vi "剖面运行流程.vi"() -> ()   [LabVIEW 2016, in "main.lvlib"]
uses:
  main.lvlib
  DAM395CF/DAM395CF.lvlib
  elevator/elevator.lvlib
  EXO2/EXO2.lvlib
  bbe/bbe.lvlib
  <vilib>/ptbypt/NI_PtbyPt.lvlib
panel:
  out "监测开始时间":timestamp
  out "编码器校准开始时间":timestamp
  out "仪器启动时间":timestamp
  out "通电时间":timestamp
  in  "bbe data":T1[](array[typedef])
  in  "EXO2 data":T2[](array[typedef])
  out "监测数据表":string[][](array[string])
  out "最深位置":dbl
  out "通知":bool
  out "Next State":string
  out "剖面路径":dbl[](array[numeric])
  out "湖面水深":dbl format="%#_6f m"
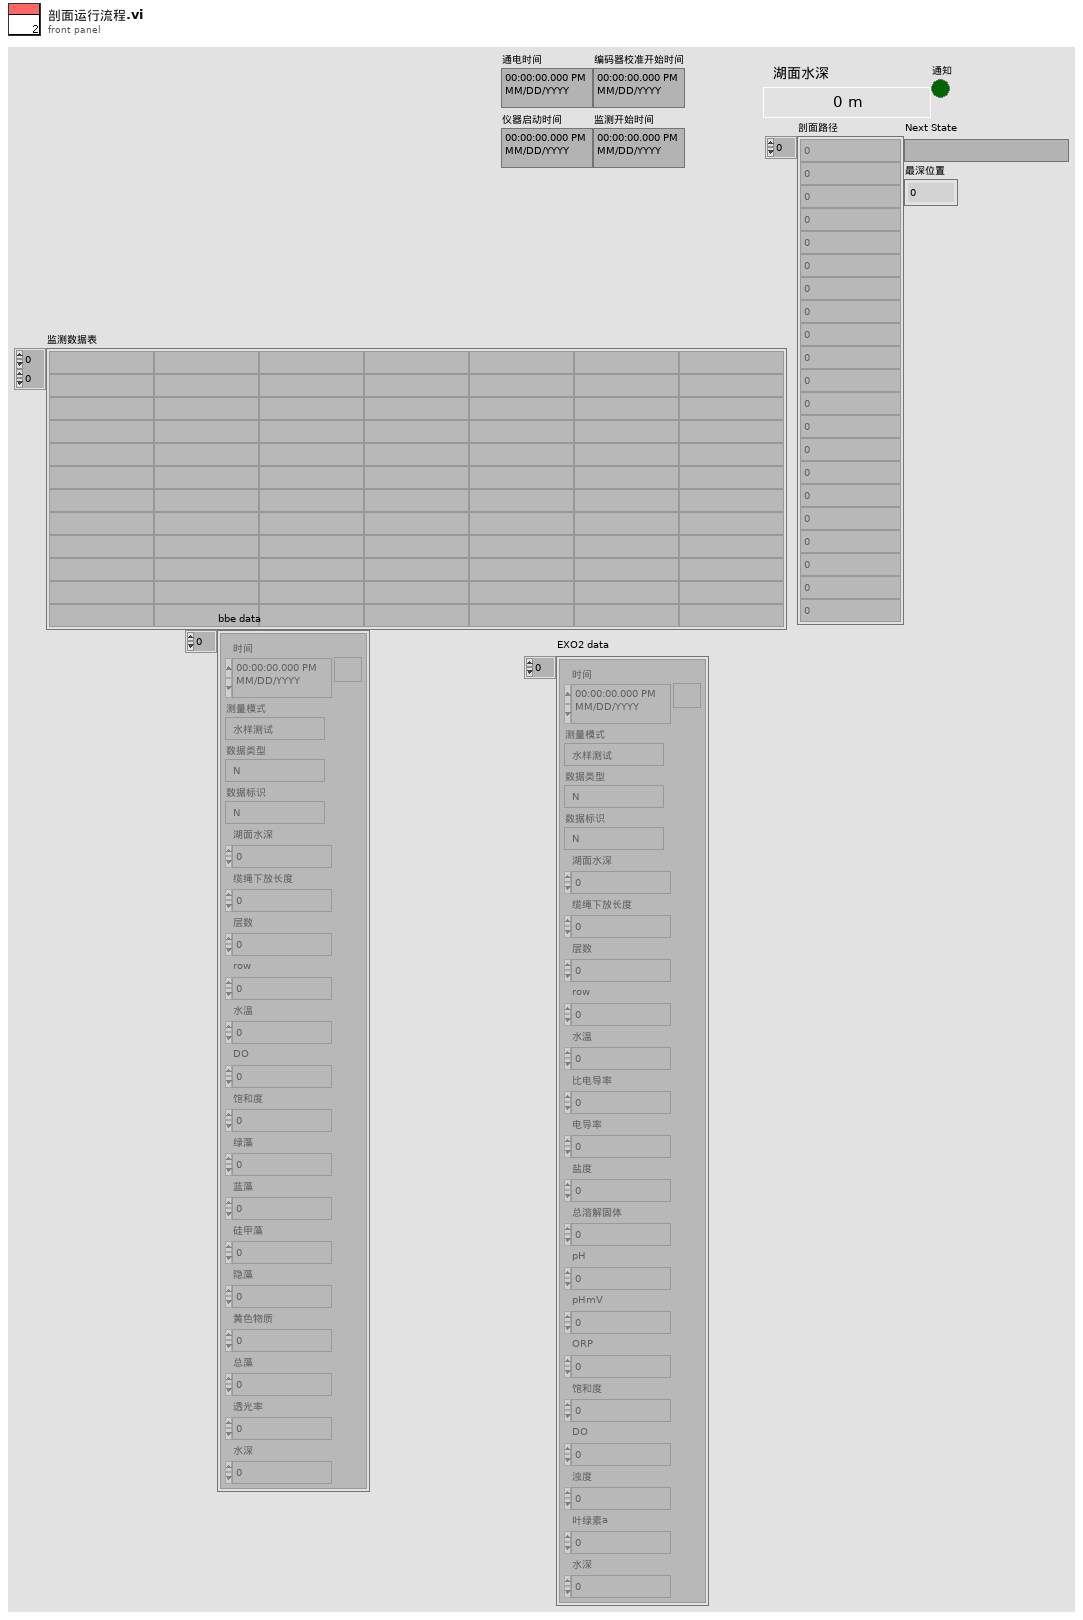
[diagram p1: front panel]
types:
  T1 = typedef "剖面数据_bbe_NAQDO.ctl" = cluster{"时间":timestamp, "测量模式":string, "数据类型":string, "数据标识":string, "湖面水深":sgl, "缆绳下放长度":sgl, "层数":u16, "row":u16, "水温":sgl, "DO":sgl, "饱和度":sgl, "绿藻":sgl, "蓝藻":sgl, "硅甲藻":sgl, "隐藻":sgl, "黄色物质":sgl, "总藻":sgl, "透光率":sgl, "水深":sgl}
  T2 = typedef "剖面数据_EXO2.ctl" = cluster{"时间":timestamp, "测量模式":string, "数据类型":string, "数据标识":string, "湖面水深":sgl, "缆绳下放长度":sgl, "层数":u16, "row":u16, "水温":sgl, "比电导率":sgl, "电导率":sgl, "盐度":sgl, "总溶解固体":sgl, "pH":sgl, "pHmV":sgl, "ORP":sgl, "饱和度":sgl, "DO":sgl, "浊度":sgl, "叶绿素a":sgl, "水深":sgl}
  T3 = enum16{"open", "poll", "close", "run", "stop", "shutdown"}
  T4 = typedef "操作日志字段定义.ctl" = cluster{"时间":timestamp, "参数":string, "日志信息":string, "流程参数":string}
  T5 = cluster{"Time":timestamp, "Temp":dbl, "SpCond":dbl, "Cond":dbl, "Sal":dbl, "TDS":dbl, "pH":dbl, "pH mV":dbl, "orp":dbl, "ODO %":dbl, "ODO mg/L":dbl, "Turb":dbl, "Chl":dbl, "Depth":dbl}
  T6 = cluster{"时间":timestamp, "Temp [℃]":dbl, "Green Algae [μg/L]":dbl, "Bluegreen [μg/L]":dbl, "Diatoms [μg/L]":dbl, "Cryptophyta [μg/L]":dbl, "Yellow substances [r.u.]":dbl, "Total Conc [μg/L]":dbl, "Transmission [%]":dbl, "Depth [m]":dbl}
  T7 = cluster{"水温":sgl, "比电导率":sgl, "电导率":sgl, "盐度":sgl, "总溶解固体":sgl, "pH":sgl, "pHmV":sgl, "ORP":sgl, "饱和度":sgl, "DO":sgl, "浊度":sgl, "叶绿素a":sgl, "水深":sgl}
  T8 = cluster{"水温":sgl, "DO":sgl, "饱和度":sgl, "绿藻":sgl, "蓝藻":sgl, "硅甲藻":sgl, "隐藻":sgl, "黄色物质":sgl, "总藻":sgl, "透光率":sgl, "水深":sgl}
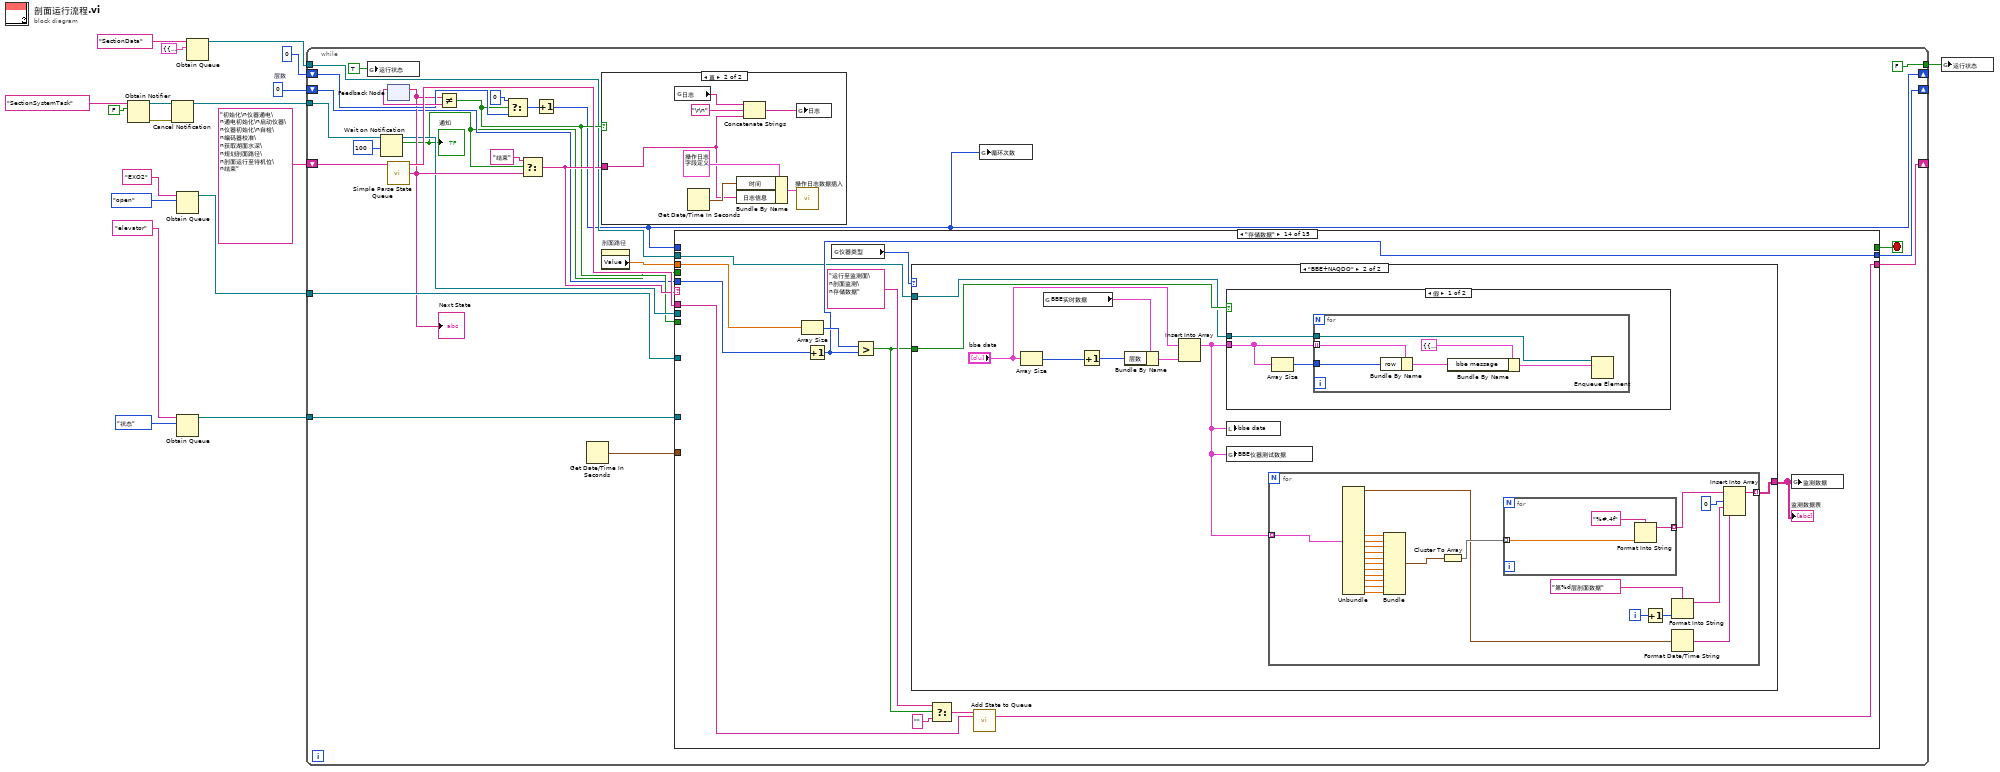
[diagram p0: block diagram]
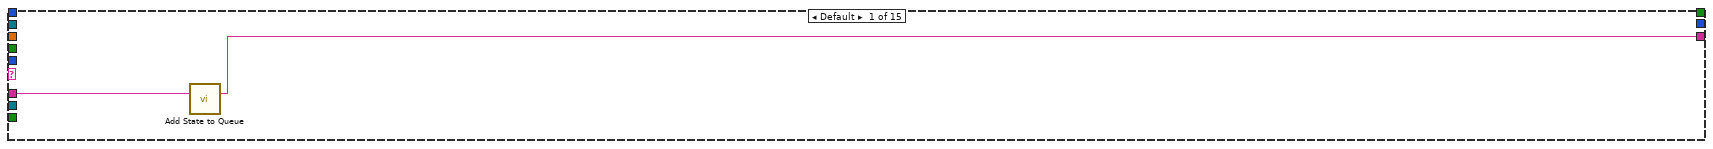
[diagram p3: hidden frame]
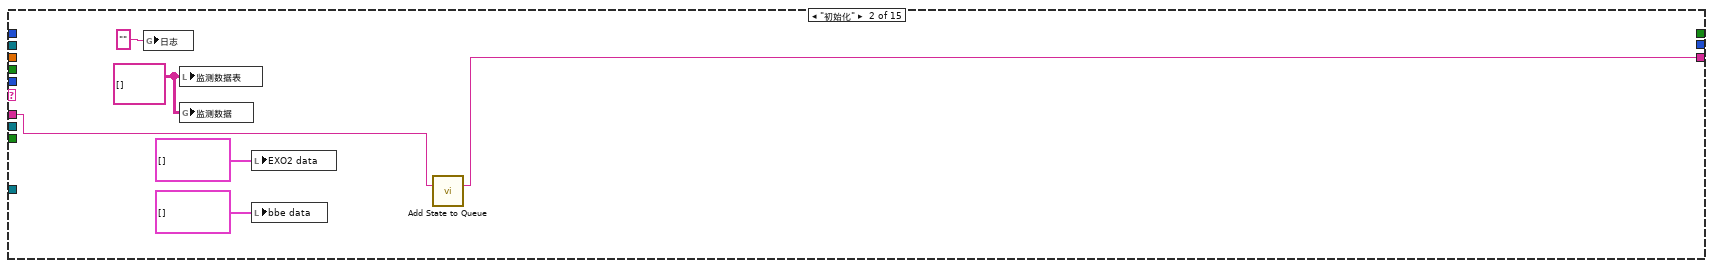
[diagram p4: hidden frame]
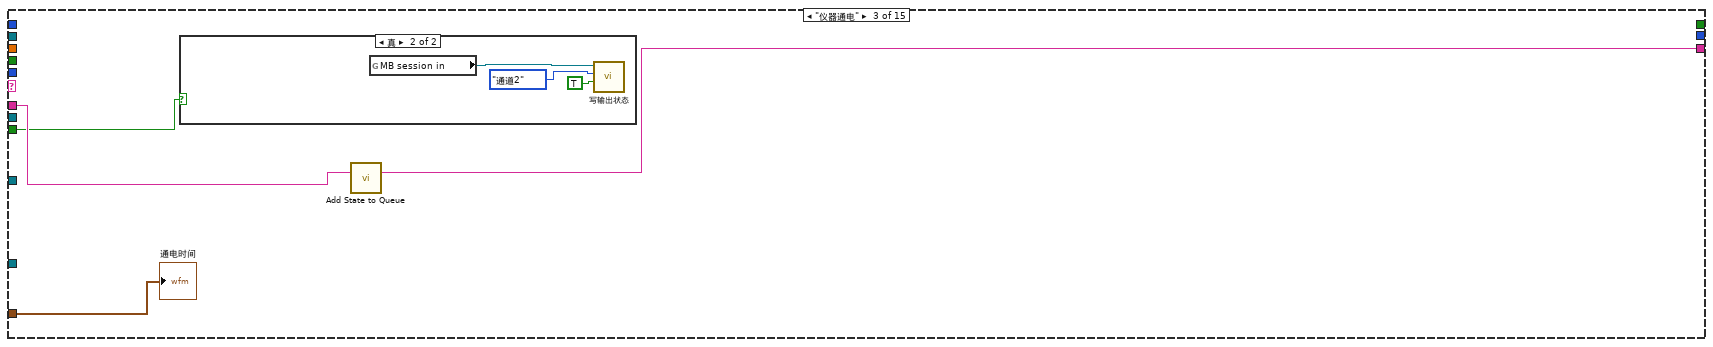
[diagram p5: hidden frame]
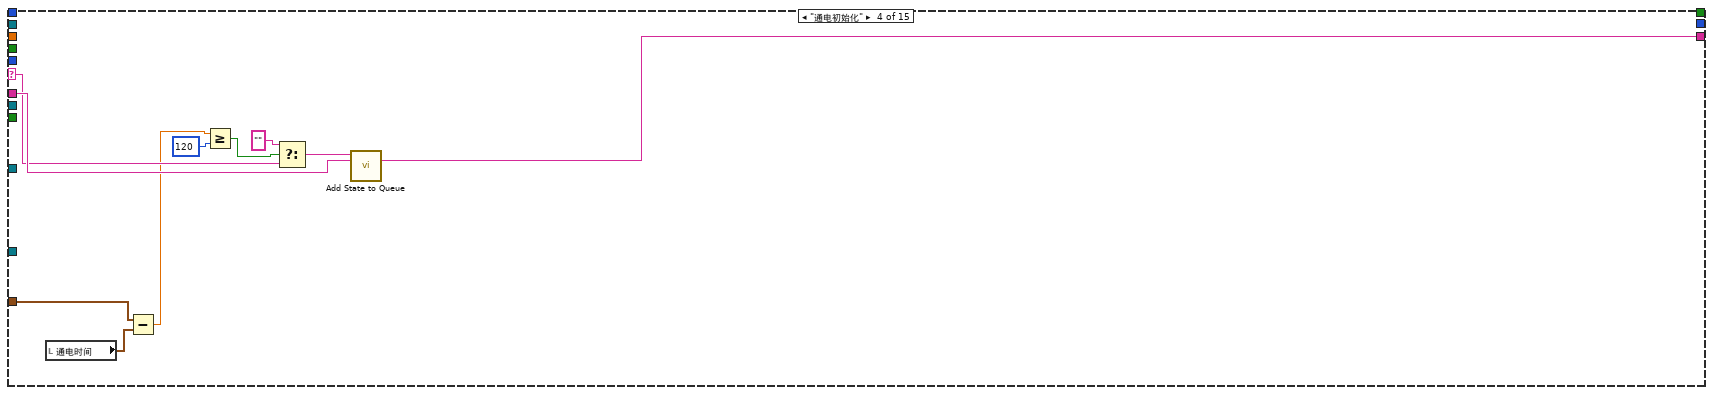
[diagram p7: hidden frame]
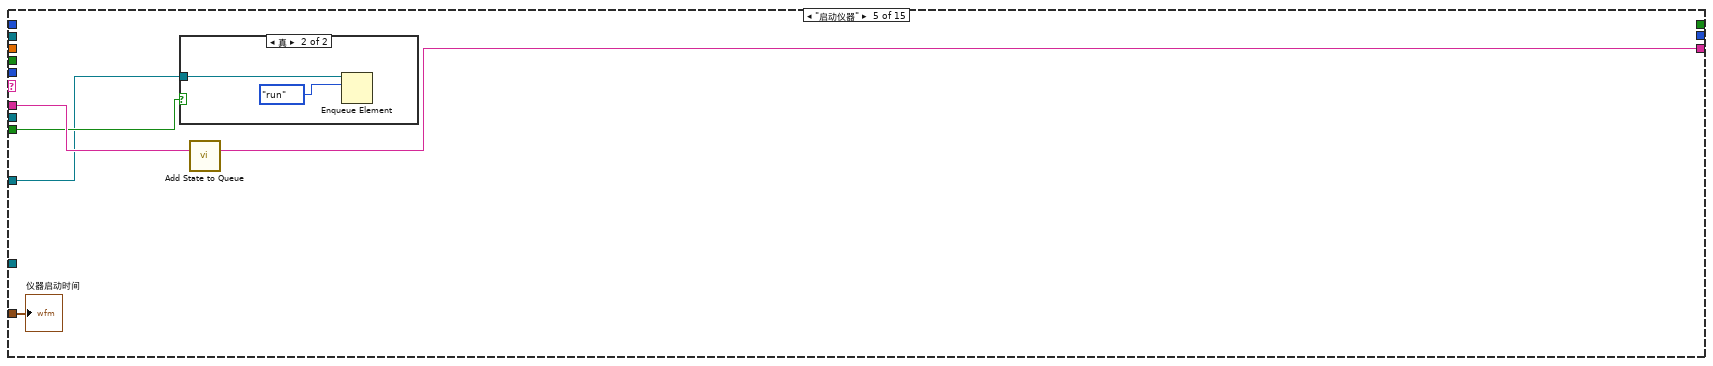
[diagram p8: hidden frame]
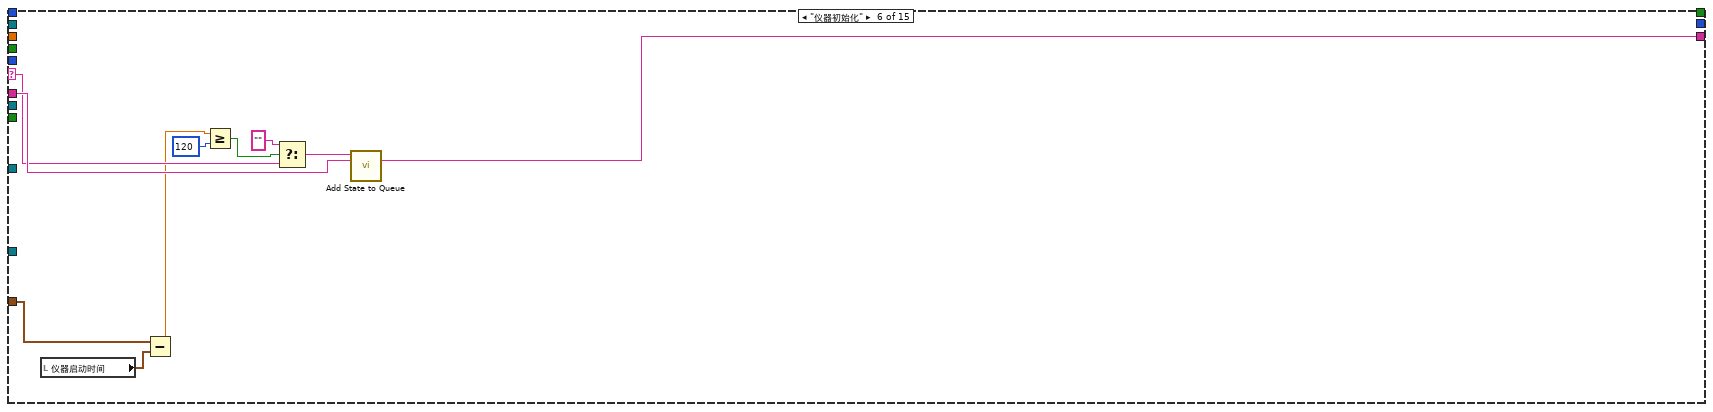
[diagram p10: hidden frame]
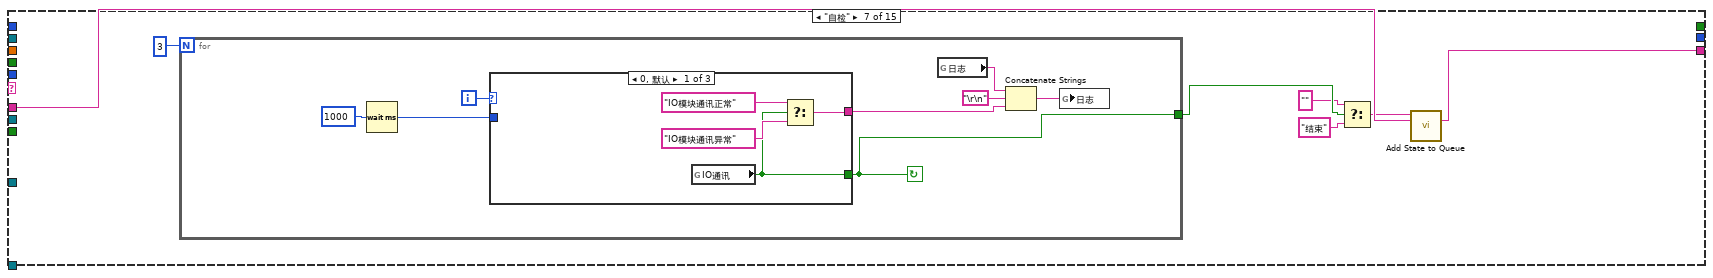
[diagram p11: hidden frame]
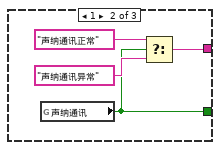
[diagram p12: hidden frame]
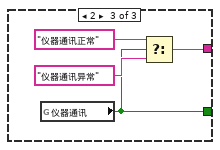
[diagram p13: hidden frame]
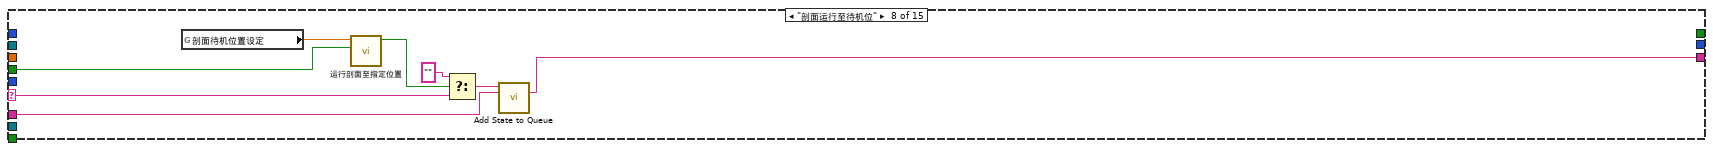
[diagram p14: hidden frame]
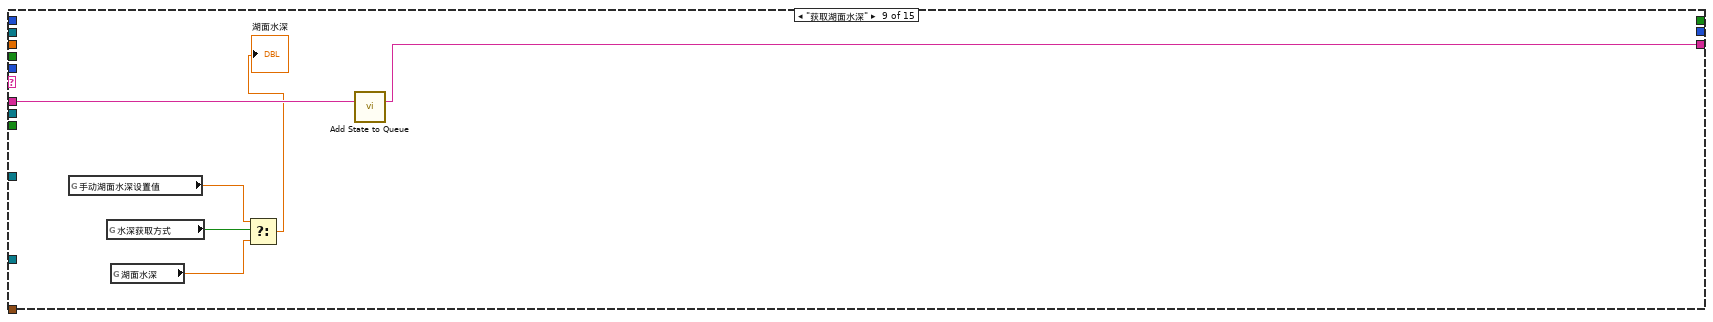
[diagram p15: hidden frame]
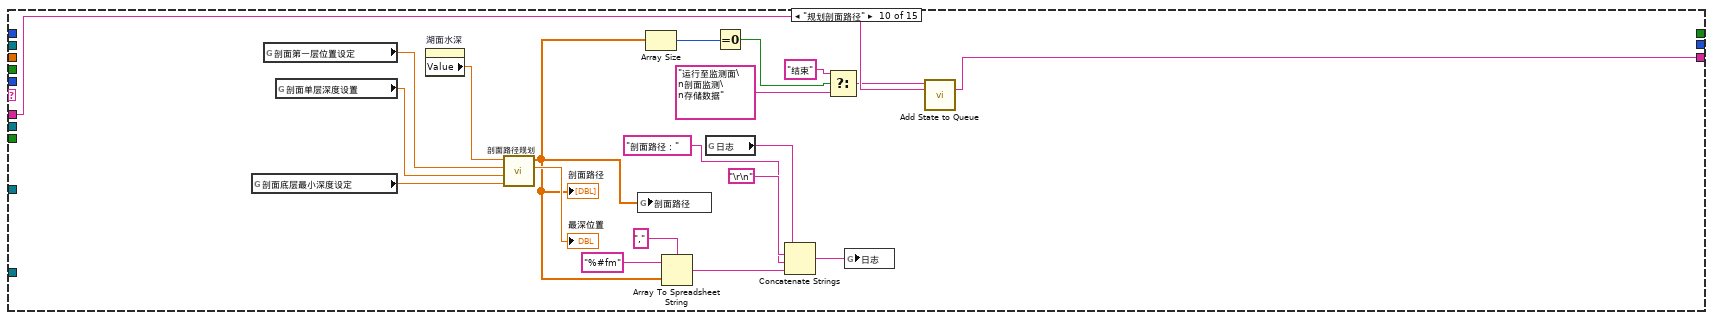
[diagram p16: hidden frame]
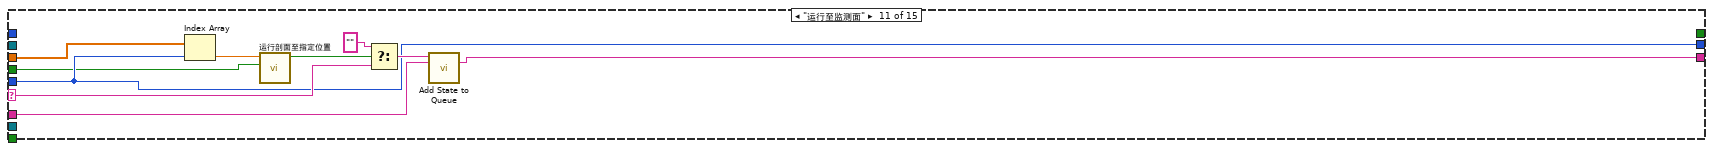
[diagram p17: hidden frame]
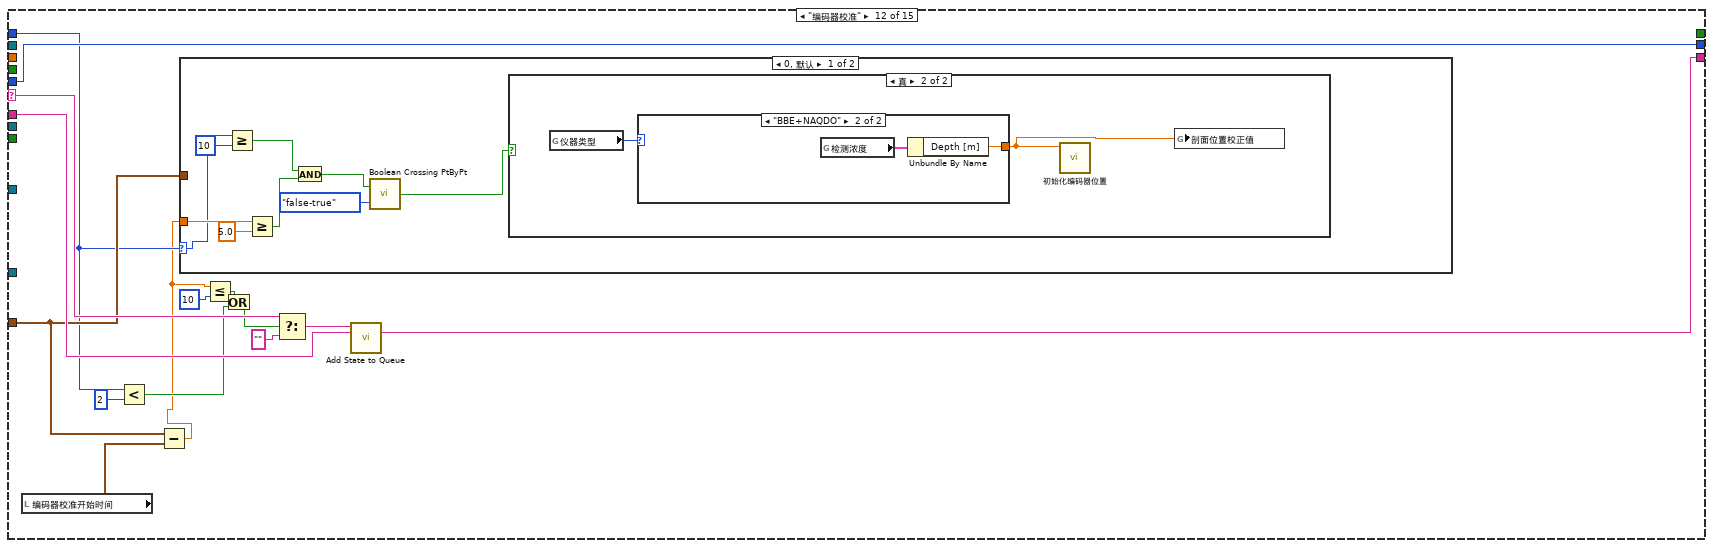
[diagram p18: hidden frame]
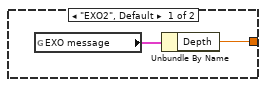
[diagram p20: hidden frame]
diagram:
  w5 = 0  # 层数
  n1 = Obtain Notifier(name (unnamed)="SectionSystemTask" ("名称（未命名）"), notification data type=FALSE) -> (notifier out=w7:refnum<notifier>, error out=w8:errorcluster)  [unwired: 2 in, 1 out]
  n2 = Cancel Notification(0:w7, 3:w8) -> (8:w6:refnum<notifier>)  [unwired: 2 out]
  n3 = Obtain Queue(name (unnamed)="EXO2" ("名称（未命名）"), element data type=T3."open" ("枚举")) -> (queue out=w12:refnum<queue>)  [unwired: 3 in, 2 out]
  n4 = Obtain Queue(name (unnamed)="elevator" ("名称（未命名）"), element data type=enum16{"状态", "上升", "下降", "停止"}."状态" ("枚举")) -> (queue out=w11:refnum<queue>)  [unwired: 3 in, 2 out]
  n5 = Obtain Queue(name (unnamed)="SectionData" ("名称（未命名）"), element data type=cluster{"EXO2 message":T2, "bbe message":T1} {"EXO2 message"={"时间"=timestamp(0 s since 1904-01-01), "测量模式"="水样测试", "数据类型"="N", "数据标识"="N", "湖面水深"=0.0, "缆绳下放长度"=0.0, "层数"=0, "row"=0, "水温"=0.0, "比电导率"=0.0, "电导率"=0.0, "盐度"=0.0, "总溶解固体"=0.0, "pH"=0.0, "pHmV"=0.0, "ORP"=0.0, "饱和度"=0.0, "DO"=0.0, "浊度"=0.0, "叶绿素a"=0.0, "水深"=0.0}, "bbe message"={"时间"=timestamp(0 s since 1904-01-01), "测量模式"="水样测试", "数据类型"="N", "数据标识"="N", "湖面水深"=0.0, "缆绳下放长度"=0.0, "层数"=0, "row"=0, "水温"=0.0, "DO"=0.0, "饱和度"=0.0, "绿藻"=0.0, "蓝藻"=0.0, "硅甲藻"=0.0, "隐藻"=0.0, "黄色物质"=0.0, "总藻"=0.0, "透光率"=0.0, "水深"=0.0}} ("簇")) -> (queue out=w2:refnum<queue>)  [unwired: 3 in, 2 out]
  n6 = while {
    shift-right: [w43] -> _
    shift-left: "初始化\n仪器通电\n通电初始化\n启动仪器\n仪器初始化\n自检\n编码器校准\n获取湖面水深\n规划剖面路径\n剖面运行至待机位\n结束" -> [w44]
    shift-right: [w20] -> _
    shift-left: 0 -> [w39]
    tunnel: w12 -> [w36]
    tunnel: w11 -> [w35]
    tunnel: w6 -> [w34]
    shift-right: [w26] -> _
    shift-left: w5 -> [w27]
    tunnel: [FALSE ("运行状态")] -> w4
    tunnel: w2 -> [w21]
    stop <- w42 stop-if-true
    n7 = global write "全局非断电保持变量.vi" "运行状态"(TRUE ("运行状态")) -> ()
    n8 = Wait on Notification(notifier=w34, timeout in ms (-1)=100 ("超时毫秒(-1)")) -> (notifier out=w30:refnum<notifier>, notification=w22:bool)  [unwired: 2 in, 2 out]
    "通知" <- w22
    n9 = feedback #1() -> (w40:string)  [unwired: 1 in]
    n10 = call "Simple Parse State Queue.vi"("State Queue"=w44) -> ("Remain States"=w41:string, "Next State"=w32:string)  [unwired: 13 in]
    "Next State" <- w32
    n11 = feedback-in #1(w32) -> ()
    n12 = Not Equal?(x=w32, y=w40) -> (x != y?=w28:bool)
    n13 = Select(t=0, s=w28, f=w39) -> (s? t:f=w38:i32)
    n14 = Select(t="结束", s=w22, f=w32) -> (s? t:f=w29:string)
    n15 = Increment(x=w38) -> (x+1=w20:i32)
    n16 = Get Date/Time In Seconds() -> (seconds since 1Jan1904=w19:timestamp)
    n17 = case shown="真" w28 {
      tunnel: w29 -> [_ w45]
      frame False {
      }
      frame True {
        n18 = global read "全局非断电保持变量.vi" "日志"() -> (w51:string)
        n19 = Get Date/Time In Seconds() -> (seconds since 1Jan1904=w48:timestamp)
        n20 = Bundle By Name(cluster=T4 {"时间"=timestamp(0 s since 1904-01-01), "参数"="剖面系统", "日志信息"="", "流程参数"=""} ("data"), "时间"=w48, "日志信息"=w45) -> (w47:T4)
        n21 = Concatenate Strings(w51, "\r\n", w45) -> (w50:string)
        n22 = global write "全局非断电保持变量.vi" "日志"(w50) -> ()
        n23 = call "操作日志数据插入.vi"("data"=w47) -> ()  [unwired: 9 in, 1 out]
      }
    }
    n24 = property on="剖面路径" class="Arr (严格)"() -> ("Value"=w25:dbl[])  [unwired: 2 in, 2 out]
    n25 = case shown="\"存储数据\"" w29 {
      selector: w29 -> [_ _ _ w72 _ w89 _ w124 _ _ w160 w174 w203 _ w318]
      tunnel: [w52 w59 w62 w75 w80 w92 w99 w127 w133 w153 w163 w178 w205 w222 w327] -> w43
      tunnel: [_ _ _ _ _ _ _ _ _ _ _ _ _ _ TRUE] -> w42
      tunnel: w41 -> [w53 w58 w63 w76 w81 w93 w100 w128 w134 w154 w164 w179 w206 w223 w325]
      tunnel: w20 -> [_ _ _ _ _ _ _ _ _ _ _ w166 _ _ _]
      tunnel: w28 -> [_ _ w61 _ w79 _ _ _ _ _ _ _ w199 _ _]
      tunnel: w36 -> [_ _ _ _ w78 _ _ _ _ _ _ _ _ _ w324]
      tunnel: w35 -> [_ _ _ _ _ _ _ _ _ _ _ _ _ _ w323]
      tunnel: w30 -> [_ _ _ _ _ _ _ _ _ _ _ _ _ _ w322]
      tunnel: w27 -> [_ _ _ _ _ _ _ _ _ _ w156 w177 w200 w216 _]
      tunnel: [_ _ _ _ _ _ _ _ _ _ w156 w177 w200 w215 _] -> w26
      tunnel: w25 -> [_ _ _ _ _ _ _ _ _ _ w157 _ _ w221 _]
      tunnel: w22 -> [_ _ _ _ _ _ _ w121 _ _ w155 _ _ _ _]
      tunnel: w21 -> [_ _ _ _ _ _ _ _ _ _ _ _ _ w211 w314]
      tunnel: w19 -> [_ _ w60 w68 w77 w85 _ _ _ _ _ w170 w198 _ _]
      frame Default {
        n26 = call "Add State to Queue.vi"("State(s) In (\"\")"=w53) -> ("States Out"=w52:string)  [unwired: 14 in]
      }
      frame "初始化" {
        w56 = string[][] [] ("添加的数组")
        n27 = global write "全局非断电保持变量.vi" "日志"("" ("日志")) -> ()
        n28 = local write "监测数据表"(w56) -> ()
        n29 = global write "全局非断电保持变量.vi" "监测数据"(w56) -> ()
        n30 = local write "EXO2 data"(T2[] [] ("EXO2 data")) -> ()
        n31 = local write "bbe data"(T1[] [] ("bbe data")) -> ()
        n32 = call "Add State to Queue.vi"("State(s) In (\"\")"=w58) -> ("States Out"=w59:string)  [unwired: 14 in]
      }
      frame "仪器通电" {
        n33 = case shown="真" w61 {
          frame False {
          }
          frame True {
            n34 = global read "elevator 全局变量.vi" "MB session in"() -> (w65:refnum<class "MB_Master.lvclass">)
            n35 = call "写输出状态.vi"("value"=TRUE, "通道"=enum16{"通道0", "通道1", "通道2", "通道3"}."通道2", "MB session in"=w65) -> ()  [unwired: 7 in, 2 out]
          }
        }
        n36 = call "Add State to Queue.vi"("State(s) In (\"\")"=w63) -> ("States Out"=w62:string)  [unwired: 14 in]
        "通电时间" <- w60
      }
      frame "通电初始化" {
        n37 = local read "通电时间"() -> (w69:timestamp)
        n38 = Subtract(x=w68, y=w69) -> (x-y=w67:dbl)
        n39 = Greater Or Equal?(x=w67, y=120) -> (x >= y?=w73:bool)
        n40 = Select(t="", s=w73, f=w72) -> (s? t:f=w71:string)
        n41 = call "Add State to Queue.vi"("State(s) In Front (\"\")"=w71, "State(s) In (\"\")"=w76) -> ("States Out"=w75:string)  [unwired: 13 in]
      }
      frame "启动仪器" {
        n42 = case shown="真" w79 {
          tunnel: w78 -> [_ w83]
          frame False {
          }
          frame True {
            n43 = Enqueue Element(queue=w83, element=T3."run" ("元素")) -> ()  [unwired: 2 in, 3 out]
          }
        }
        n44 = call "Add State to Queue.vi"("State(s) In (\"\")"=w81) -> ("States Out"=w80:string)  [unwired: 14 in]
        "仪器启动时间" <- w77
      }
      frame "仪器初始化" {
        n45 = local read "仪器启动时间"() -> (w86:timestamp)
        n46 = Subtract(x=w85, y=w86) -> (x-y=w84:dbl)
        n47 = Greater Or Equal?(x=w84, y=120) -> (x >= y?=w90:bool)
        n48 = Select(t="", s=w90, f=w89) -> (s? t:f=w88:string)
        n49 = call "Add State to Queue.vi"("State(s) In Front (\"\")"=w88, "State(s) In (\"\")"=w93) -> ("States Out"=w92:string)  [unwired: 13 in]
      }
      frame "自检" {
        n50 = for {
          N: 3 -> [_]
          tunnel: [w102] -> w97
          i -> [w107]
          stop <- w102 continue-if-true
          n51 = Wait (ms)(milliseconds to wait=u32 1000 ("等待时间（毫秒）")) -> (millisecond timer value=w101:u32)
          n52 = case shown="0, 默认" w107 {
            tunnel: [w111 w115 w119] -> w103
            tunnel: [w109 w113 w117] -> w102
            tunnel: w101 -> [_ _ _]
            frame 0, Default {
              n53 = global read "全局非断电保持变量.vi" "IO通讯"() -> (w109:bool)
              n54 = Select(t="IO模块通讯正常", s=w109, f="IO模块通讯异常") -> (s? t:f=w111:string)
            }
            frame 1 {
              n55 = global read "全局非断电保持变量.vi" "声纳通讯"() -> (w113:bool)
              n56 = Select(t="声纳通讯正常", s=w113, f="声纳通讯异常") -> (s? t:f=w115:string)
            }
            frame 2 {
              n57 = global read "全局非断电保持变量.vi" "仪器通讯"() -> (w117:bool)
              n58 = Select(t="仪器通讯正常", s=w117, f="仪器通讯异常") -> (s? t:f=w119:string)
            }
          }
          n59 = global read "全局非断电保持变量.vi" "日志"() -> (w104:string)
          n60 = Concatenate Strings(w104, "\r\n", w103) -> (w105:string)
          n61 = global write "全局非断电保持变量.vi" "日志"(w105) -> ()
        }
        n62 = Select(t="", s=w97, f="结束") -> (s? t:f=w95:string)
        n63 = call "Add State to Queue.vi"("State(s) In Front (\"\")"=w95, "State(s) In (\"\")"=w100) -> ("States Out"=w99:string)  [unwired: 13 in]
      }
      frame "剖面运行至待机位" {
        n64 = global read "全局断电保存变量.vi" "剖面待机位置设定"() -> (w126:dbl)
        n65 = call "运行剖面至指定位置.vi"("停止"=w121, "位置设置值"=w126) -> ("定位完成"=w125:bool)  [unwired: 8 in, 1 out]
        n66 = Select(t="", s=w125, f=w124) -> (s? t:f=w123:string)
        n67 = call "Add State to Queue.vi"("State(s) In Front (\"\")"=w123, "State(s) In (\"\")"=w128) -> ("States Out"=w127:string)  [unwired: 13 in]
      }
      frame "获取湖面水深" {
        n68 = global read "全局断电保存变量.vi" "手动湖面水深设置值"() -> (w131:sgl)
        n69 = global read "全局断电保存变量.vi" "水深获取方式"() -> (w132:bool)
        n70 = global read "全局非断电保持变量.vi" "湖面水深"() -> (w130:dbl)
        n71 = Select(t=w131, s=w132, f=w130) -> (s? t:f=→"湖面水深":dbl)
        n72 = call "Add State to Queue.vi"("State(s) In (\"\")"=w134) -> ("States Out"=w133:string)  [unwired: 14 in]
      }
      frame "规划剖面路径" {
        n73 = global read "全局断电保存变量.vi" "剖面底层最小深度设定"() -> (w149:dbl)
        n74 = global read "全局断电保存变量.vi" "剖面第一层位置设定"() -> (w151:dbl)
        n75 = global read "全局断电保存变量.vi" "剖面单层深度设置"() -> (w150:dbl)
        n76 = property on="湖面水深" class="DigNum (严格)"() -> ("Value"=w152:dbl)  [unwired: 2 in, 2 out]
        n77 = call "剖面路径规划.vi"("剖面底层最小深度设定"=w149, "剖面单层深度设置"=w150, "剖面第一层位置设定"=w151, "水深"=w152) -> ("最深位置"=→"最深位置":dbl, "剖面路径"=w140:dbl[])  [unwired: 5 in, 1 out]
        "剖面路径" <- w140
        n78 = global write "全局非断电保持变量.vi" "剖面路径"(w140) -> ()
        n79 = Array Size(array=w140) -> (size(s)=w139:i32)
        n80 = Array To Spreadsheet String(delimiter (Tab)="," ("分隔符(Tab)"), array=w140, 3:"%#fm" ("格式字符串")) -> (spreadsheet string=w142:string)
        n81 = global read "全局非断电保持变量.vi" "日志"() -> (w145:string)
        n82 = Equal To 0?(x=w139) -> (x = 0?=w138:bool)
        n83 = Concatenate Strings(w145, "\r\n", "剖面路径：" ("字符串"), w142) -> (w146:string)
        n84 = Select(t="结束", s=w138, f="运行至监测面\n剖面监测\n存储数据") -> (s? t:f=w135:string)
        n85 = global write "全局非断电保持变量.vi" "日志"(w146) -> ()
        n86 = call "Add State to Queue.vi"("State(s) In Front (\"\")"=w135, "State(s) In (\"\")"=w154) -> ("States Out"=w153:string)  [unwired: 13 in]
      }
      frame "运行至监测面" {
        n87 = Index Array(array=w157, index=w156) -> (element=w162:dbl)
        n88 = call "运行剖面至指定位置.vi"("停止"=w155, "位置设置值"=w162) -> ("定位完成"=w161:bool)  [unwired: 8 in, 1 out]
        n89 = Select(t="", s=w161, f=w160) -> (s? t:f=w159:string)
        n90 = call "Add State to Queue.vi"("State(s) In Front (\"\")"=w159, "State(s) In (\"\")"=w164) -> ("States Out"=w163:string)  [unwired: 13 in]
      }
      frame "编码器校准" {
        n91 = local read "编码器校准开始时间"() -> (w171:timestamp)
        n92 = Less?(x=w166, y=2) -> (x < y?=w167:bool)
        n93 = Subtract(x=w170, y=w171) -> (x-y=w165:dbl)
        n94 = case shown="0, 默认" w166 {
          selector: w166 -> [w186 _]
          tunnel: w170 -> [_ w195]
          tunnel: w165 -> [w188 _]
          frame 0, Default {
            n95 = Greater Or Equal?(x=w186, y=10) -> (x >= y?=w183:bool)
            n96 = Greater Or Equal?(x=w188, y=5.0) -> (x >= y?=w184:bool)
            n97 = And(x=w183, y=w184) -> (x .and. y?=w182:bool)
            n98 = call <vilib>:"Boolean Crossing PtByPt.vi"("direction"=enum16{"either", "false-true", "true-false"}."false-true", "input"=w182) -> ("crossing"=w181:bool)  [unwired: 1 in]
            n99 = case shown="真" w181 {
              frame False {
              }
              frame True {
                n100 = global read "全局断电保存变量.vi" "仪器类型"() -> (w189:enum16{"EXO2", "BBE+NAQDO"})
                n101 = case shown="\"BBE+NAQDO\"" w189 {
                  tunnel: [w192 w193] -> w190
                  frame "EXO2", Default {
                    n102 = global read "EXO2全局变量.vi" "EXO message"() -> (w191:T5)
                    n103 = Unbundle By Name(w191) -> ("Depth"=w192:dbl)
                  }
                  frame "BBE+NAQDO" {
                    n104 = global read "过程变量.vi" "检测浓度"() -> (w194:T6)
                    n105 = Unbundle By Name(w194) -> ("Depth [m]"=w193:dbl)
                  }
                }
                n106 = call "初始化编码器位置.vi"("原始位置"=w190) -> ()  [unwired: 10 in, 1 out]
                n107 = global write "全局断电保存变量.vi" "剖面位置校正值"(w190) -> ()
              }
            }
          }
          frame 1 {
            "编码器校准开始时间" <- w195
          }
        }
        n108 = Less Or Equal?(x=w165, y=10) -> (x <= y?=w175:bool)
        n109 = Or(x=w175, y=w167) -> (x .or. y?=w168:bool)
        n110 = Select(t=w174, s=w168, f="") -> (s? t:f=w173:string)
        n111 = call "Add State to Queue.vi"("State(s) In Front (\"\")"=w173, "State(s) In (\"\")"=w179) -> ("States Out"=w178:string)  [unwired: 13 in]
      }
      frame "剖面监测" {
        n112 = case shown="假" w199 {
          tunnel: w198 -> [w209 w210]
          tunnel: [w207 _] -> w196
          frame False {
            n113 = local read "监测开始时间"() -> (w208:timestamp)
            n114 = Subtract(x=w209, y=w208) -> (x-y=w207:dbl)
          }
          frame True {
            "监测开始时间" <- w210
          }
        }
        n115 = global read "全局断电保存变量.vi" "单层监测时间"() -> (w197:u16)
        n116 = Greater Or Equal?(x=w196, y=w197) -> (x >= y?=w204:bool)
        n117 = Select(t="", s=w204, f=w203) -> (s? t:f=w202:string)
        n118 = call "Add State to Queue.vi"("State(s) In Front (\"\")"=w202, "State(s) In (\"\")"=w206) -> ("States Out"=w205:string)  [unwired: 13 in]
      }
      frame "存储数据" {
        n119 = Array Size(array=w221) -> (size(s)=w220:i32)
        n120 = Increment(x=w216) -> (x+1=w215:i32)
        n121 = global read "全局断电保存变量.vi" "仪器类型"() -> (w212:enum16{"EXO2", "BBE+NAQDO"})
        n122 = Greater?(x=w220, y=w215) -> (0:w214:bool)
        n123 = case shown="\"BBE+NAQDO\"" w212 {
          tunnel: w214 -> [w232 w278]
          tunnel: [w231 w277] -> w213
          tunnel: w211 -> [w230 w273]
          frame "EXO2", Default {
            n124 = Array Size(array="EXO2 data") -> (size(s)=w227:i32)
            n125 = global read "全局非断电保持变量.vi" "EXO2实时数据"() -> (w225:T2)
            n126 = Increment(x=w227) -> (x+1=w224:i32)
            n127 = Bundle By Name(cluster=w225, "层数"=w224) -> (w229:T2)
            n128 = Insert Into Array(array="EXO2 data", new element=w229) -> (w226:T2[])  [unwired: 1 in]
            n129 = local write "EXO2 data"(w226) -> ()
            n130 = global write "全局非断电保持变量.vi" "EXO2仪器测试数据"(w226) -> ()
            n131 = case shown="假" w232 {
              tunnel: w230 -> [w263 _]
              tunnel: w226 -> [w261 _]
              frame False {
                n132 = Array Size(array=w261) -> (size(s)=w262:i32)
                n133 = for {
                  tunnel: w263 -> [w269]
                  tunnel: w261 -> [w266] mode=indexing
                  tunnel: w262 -> [w264]
                  n134 = Bundle By Name(cluster=w266, "row"=w264) -> (w265:T2)
                  n135 = Bundle By Name(cluster=cluster{"EXO2 message":T2, "bbe message":T1} {"EXO2 message"={"时间"=timestamp(0 s since 1904-01-01), "测量模式"="", "数据类型"="", "数据标识"="", "湖面水深"=0.0, "缆绳下放长度"=0.0, "层数"=0, "row"=0, "水温"=0.0, "比电导率"=0.0, "电导率"=0.0, "盐度"=0.0, "总溶解固体"=0.0, "pH"=0.0, "pHmV"=0.0, "ORP"=0.0, "饱和度"=0.0, "DO"=0.0, "浊度"=0.0, "叶绿素a"=0.0, "水深"=0.0}, "bbe message"={"时间"=timestamp(0 s since 1904-01-01), "测量模式"="", "数据类型"="", "数据标识"="", "湖面水深"=0.0, "缆绳下放长度"=0.0, "层数"=0, "row"=0, "水温"=0.0, "DO"=0.0, "饱和度"=0.0, "绿藻"=0.0, "蓝藻"=0.0, "硅甲藻"=0.0, "隐藻"=0.0, "黄色物质"=0.0, "总藻"=0.0, "透光率"=0.0, "水深"=0.0}} ("元素"), "EXO2 message"=w265) -> (w267:cluster{"EXO2 message":T2, "bbe message":T1})
                  n136 = Enqueue Element(queue=w269, element=w267) -> ()  [unwired: 2 in, 3 out]
                }
              }
              frame True {
              }
            }
            n137 = for {
              tunnel: [w248] -> w231 mode=indexing
              tunnel: w226 -> [w242] mode=indexing
              i -> [w245]
              n138 = Unbundle(w242) -> ("时间"=w251:timestamp, "水温"=w256:sgl, "比电导率"=w257:sgl, "电导率"=w255:sgl, "盐度"=w254:sgl, "总溶解固体"=w253:sgl, "pH"=w252:sgl, "pHmV"=w241:sgl, "ORP"=w240:sgl, "饱和度"=w239:sgl, "DO"=w238:sgl, "浊度"=w236:sgl, "叶绿素a"=w237:sgl, "水深"=w233:sgl)  [unwired: 7 out]
              n139 = Bundle("水温"=w256, "比电导率"=w257, "电导率"=w255, "盐度"=w254, "总溶解固体"=w253, "pH"=w252, "pHmV"=w241, "ORP"=w240, "饱和度"=w239, "DO"=w238, "浊度"=w236, "叶绿素a"=w237, "水深"=w233) -> (w235:T7)  [unwired: 1 in]
              n140 = Cluster To Array(cluster=w235) -> (array=w234:sgl[])
              n141 = for {
                tunnel: [w259] -> w250 mode=indexing
                tunnel: w234 -> [w258] mode=indexing
                n142 = Format Into String(format string="%#.4f" ("格式字符串"), w258) -> (resulting string=w259:string)  [unwired: 2 in, 1 out]
              }
              n143 = Increment(x=w245) -> (x+1=w244:i32)
              n144 = Format Into String(format string="第%d层剖面数据" ("格式字符串"), w244) -> (resulting string=w243:string)  [unwired: 2 in, 1 out]
              n145 = Format Date/Time String(seconds (now)=w251) -> (date/time string=w249:string)  [unwired: 2 in]
              n146 = Insert Into Array(array=w250, index=0 ("索引"), new element #1=w243, new element #2=w249) -> (w248:string[])
            }
          }
          frame "BBE+NAQDO" {
            n147 = Array Size(array="bbe data") -> (size(s)=w274:i32)
            n148 = global read "全局非断电保持变量.vi" "BBE实时数据"() -> (w271:T1)
            n149 = Increment(x=w274) -> (x+1=w270:i32)
            n150 = Bundle By Name(cluster=w271, "层数"=w270) -> (w276:T1)
            n151 = Insert Into Array(array="bbe data", new element=w276) -> (w272:T1[])  [unwired: 1 in]
            n152 = case shown="假" w278 {
              tunnel: w272 -> [w306 _]
              tunnel: w273 -> [w307 _]
              frame False {
                n153 = Array Size(array=w306) -> (size(s)=w305:i32)
                n154 = for {
                  tunnel: w306 -> [w311] mode=indexing
                  tunnel: w307 -> [w310]
                  tunnel: w305 -> [w308]
                  n155 = Bundle By Name(cluster=w311, "row"=w308) -> (w309:T1)
                  n156 = Bundle By Name(cluster=cluster{"EXO2 message":T2, "bbe message":T1} {"EXO2 message"={"时间"=timestamp(0 s since 1904-01-01), "测量模式"="", "数据类型"="", "数据标识"="", "湖面水深"=0.0, "缆绳下放长度"=0.0, "层数"=0, "row"=0, "水温"=0.0, "比电导率"=0.0, "电导率"=0.0, "盐度"=0.0, "总溶解固体"=0.0, "pH"=0.0, "pHmV"=0.0, "ORP"=0.0, "饱和度"=0.0, "DO"=0.0, "浊度"=0.0, "叶绿素a"=0.0, "水深"=0.0}, "bbe message"={"时间"=timestamp(0 s since 1904-01-01), "测量模式"="", "数据类型"="", "数据标识"="", "湖面水深"=0.0, "缆绳下放长度"=0.0, "层数"=0, "row"=0, "水温"=0.0, "DO"=0.0, "饱和度"=0.0, "绿藻"=0.0, "蓝藻"=0.0, "硅甲藻"=0.0, "隐藻"=0.0, "黄色物质"=0.0, "总藻"=0.0, "透光率"=0.0, "水深"=0.0}} ("元素"), "bbe message"=w309) -> (w312:cluster{"EXO2 message":T2, "bbe message":T1})
                  n157 = Enqueue Element(queue=w310, element=w312) -> ()  [unwired: 2 in, 3 out]
                }
              }
              frame True {
              }
            }
            n158 = local write "bbe data"(w272) -> ()
            n159 = global write "全局非断电保持变量.vi" "BBE仪器测试数据"(w272) -> ()
            n160 = for {
              tunnel: w272 -> [w301] mode=indexing
              tunnel: [w295] -> w277 mode=indexing
              i -> [w292]
              n161 = Unbundle(w301) -> ("时间"=w298:timestamp, "水温"=w282:sgl, "DO"=w283:sgl, "饱和度"=w284:sgl, "绿藻"=w285:sgl, "蓝藻"=w286:sgl, "硅甲藻"=w287:sgl, "隐藻"=w288:sgl, "黄色物质"=w289:sgl, "总藻"=w281:sgl, "透光率"=w280:sgl, "水深"=w279:sgl)  [unwired: 7 out]
              n162 = Bundle("水温"=w282, "DO"=w283, "饱和度"=w284, "绿藻"=w285, "蓝藻"=w286, "硅甲藻"=w287, "隐藻"=w288, "黄色物质"=w289, "总藻"=w281, "透光率"=w280, "水深"=w279) -> (w300:T8)  [unwired: 1 in]
              n163 = Cluster To Array(cluster=w300) -> (array=w299:sgl[])
              n164 = for {
                tunnel: w299 -> [w304] mode=indexing
                tunnel: [w302] -> w297 mode=indexing
                n165 = Format Into String(format string="%#.4f" ("格式字符串"), w304) -> (resulting string=w302:string)  [unwired: 2 in, 1 out]
              }
              n166 = Increment(x=w292) -> (x+1=w291:i32)
              n167 = Format Into String(format string="第%d层剖面数据" ("格式字符串"), w291) -> (resulting string=w290:string)  [unwired: 2 in, 1 out]
              n168 = Format Date/Time String(seconds (now)=w298) -> (date/time string=w296:string)  [unwired: 2 in]
              n169 = Insert Into Array(array=w297, index=0 ("索引"), new element #1=w290, new element #2=w296) -> (w295:string[])
            }
          }
        }
        "监测数据表" <- w213
        n170 = Select(t="运行至监测面\n剖面监测\n存储数据", s=w214, f="") -> (s? t:f=w218:string)
        n171 = call "Add State to Queue.vi"("State(s) In Front (\"\")"=w218, "State(s) In (\"\")"=w223) -> ("States Out"=w222:string)  [unwired: 13 in]
        n172 = global write "全局非断电保持变量.vi" "监测数据"(w213) -> ()
      }
      frame "结束" {
        n173 = Release Queue(queue=w314) -> ()  [unwired: 2 in, 3 out]
        n174 = Release Notifier(notifier=w322) -> ()  [unwired: 2 in, 3 out]
        n175 = Release Queue(queue=w324) -> ()  [unwired: 2 in, 3 out]
        n176 = Release Queue(queue=w323) -> ()  [unwired: 2 in, 3 out]
        n177 = global read "全局非断电保持变量.vi" "日志"() -> (w319:string)
        n178 = Concatenate Strings(w319, "\r\n", w318) -> (w320:string)
        n179 = global read "elevator 全局变量.vi" "MB session in"() -> (w316:refnum<class "MB_Master.lvclass">)
        n180 = global write "全局非断电保持变量.vi" "日志"(w320) -> ()
        n181 = call "写输出状态.vi"("value"=FALSE, "通道"=enum16{"通道0", "通道1", "通道2", "通道3"}."通道2", "MB session in"=w316) -> ()  [unwired: 7 in, 2 out]
        n182 = call "Add State to Queue.vi"("State(s) In (\"\")"=w325) -> ("States Out"=w327:string)  [unwired: 14 in]
        n183 = call "剖面停止.vi"() -> ()  [unwired: 11 in, 1 out]
      }
    }
    n184 = global write "全局非断电保持变量.vi" "循环次数"(w20) -> ()
  }
  n185 = global write "全局非断电保持变量.vi" "运行状态"(w4) -> ()
